vi "CaseMonitor__slk_mt.vi"() -> ()   [LabVIEW 2012, in "Lazyboots Menu Tool.lvlib"]
doc: "This VI is the core of <b>Case Monitor</b> function, and will be called by corresponding menu launcher."
uses:
  Library/Lazyboots Menu Tool.lvlib
  Private/CaseMonitor/Class/TreeView/TreeView__slk_mt.lvclass
  Private/CaseMonitor/Class/CaseModel/CaseModel__slk_mt.lvclass
  Private/CaseMonitor/Class/DatatypeAdapter/DatatypeAdapter__slk_mt.lvclass
  <vilib>/Utility/config.llb/NI_LVConfig.lvlib
panel:
  in  "Case Frames Tree":string(tree)
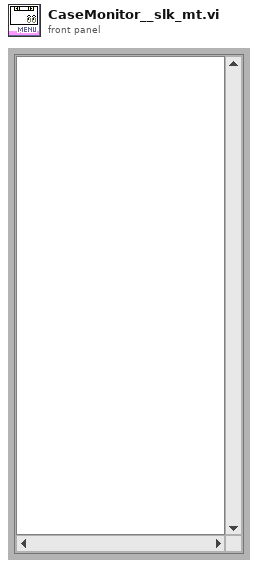
[diagram p1: front panel]
types:
  T1 = enum32{"Invalid", "Standard", "Closed", "Hidden", "Minimized", "Maximized"}
  T2 = cluster{"ItemTag":string, "OldFrame":string, "NewFrame":string}
  T3 = cluster{"Application Refnum":refnum<vi>, "VI Name":string}
  T4 = typedef "NI_LVConfig.lvlib/Config Data RefNum.ctl" = refnum<k1>
  T5 = typedef "Lazyboots Menu Tool.lvlib/TypeDef_CaseMonitorConfigure__slk_mt.ctl" = cluster{"Parent Symbol":string}
  T6 = typedef "LVPoint32TypeDef.ctl" = cluster{"Horizontal":i32, "Vertical":i32}
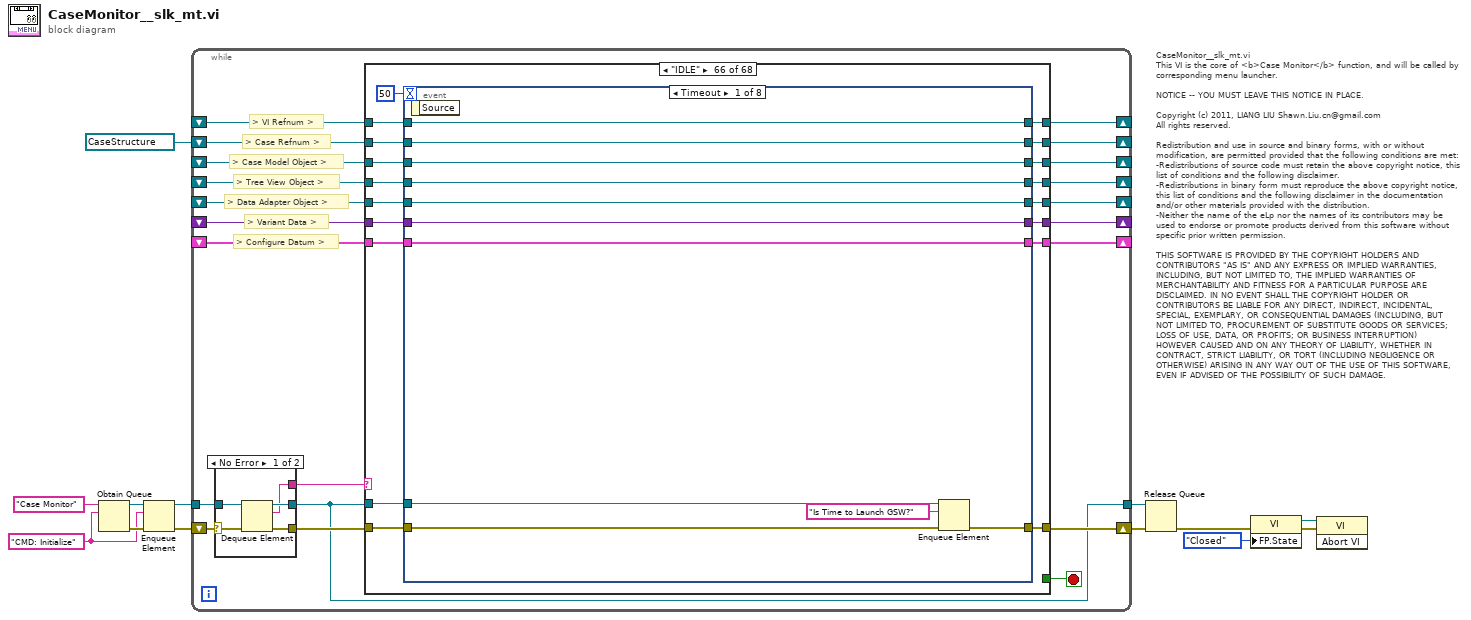
[diagram p0: block diagram]
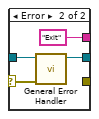
[diagram p2: hidden frame]
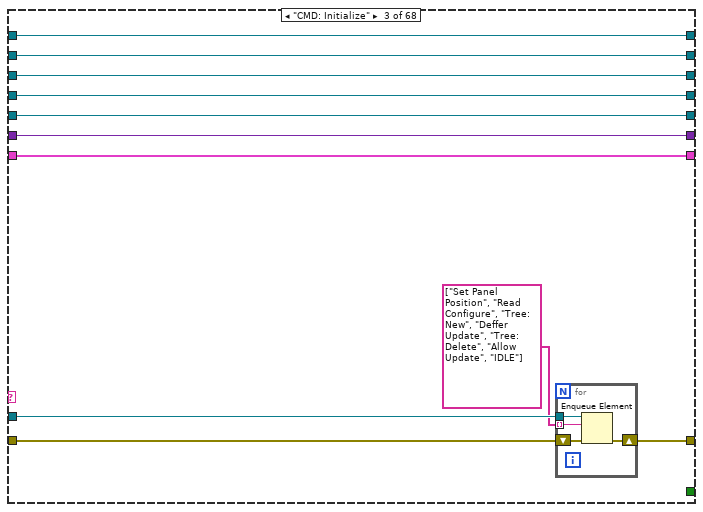
[diagram p5: hidden frame]
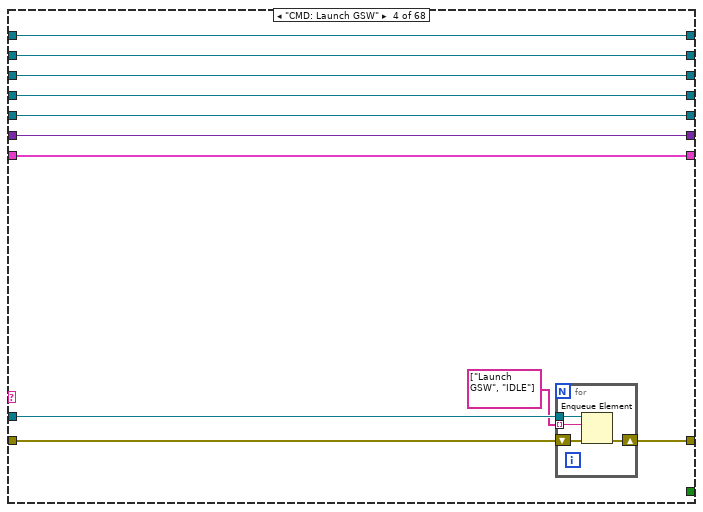
[diagram p6: hidden frame]
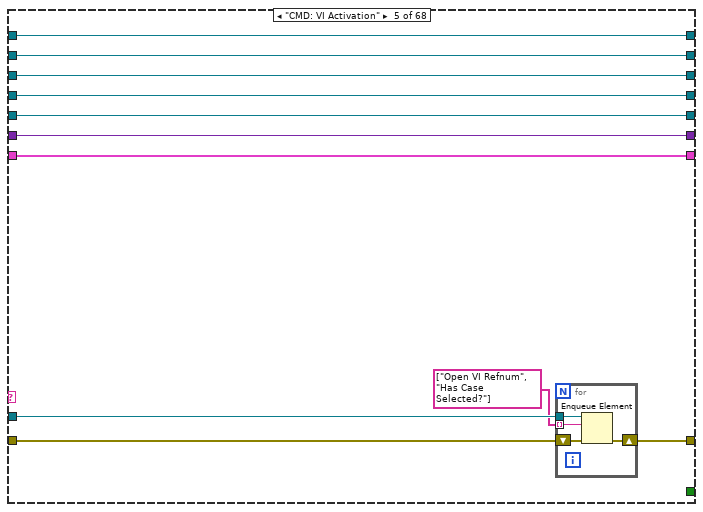
[diagram p7: hidden frame]
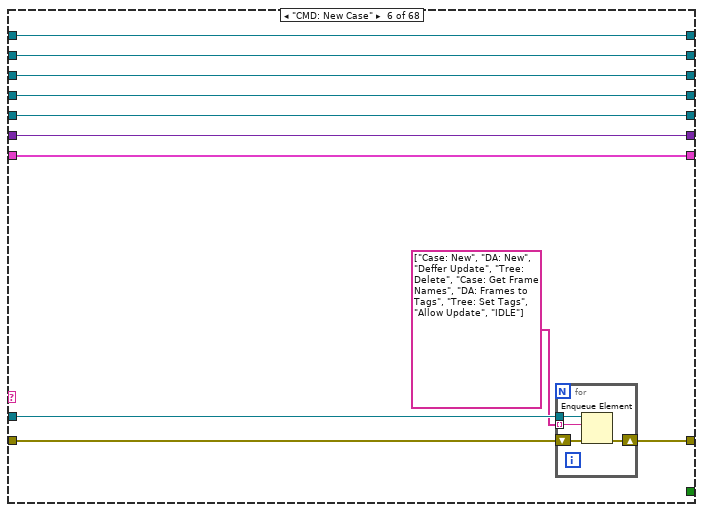
[diagram p8: hidden frame]
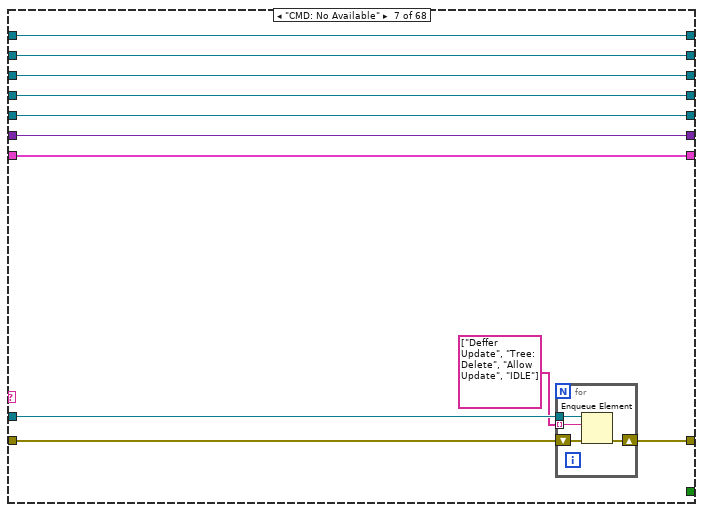
[diagram p9: hidden frame]
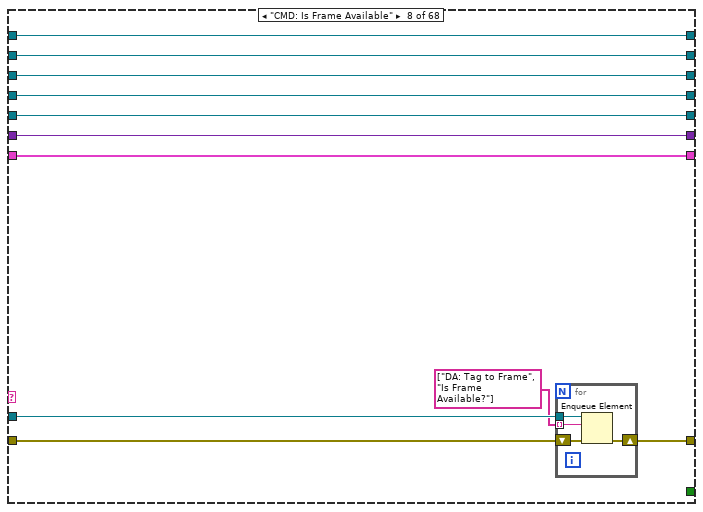
[diagram p10: hidden frame]
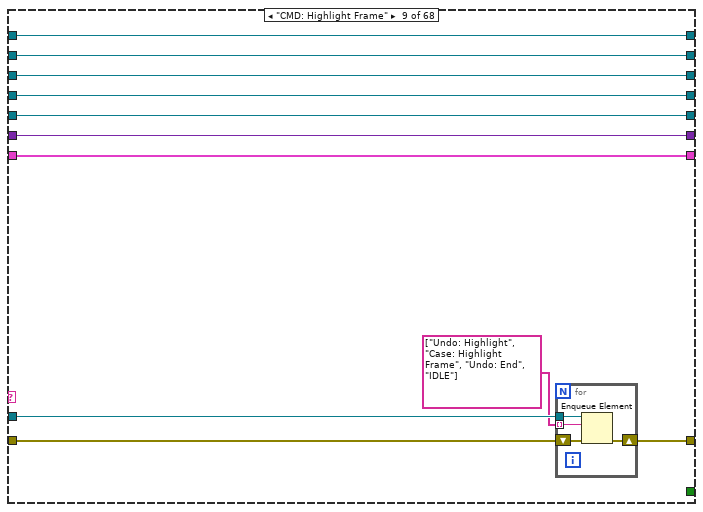
[diagram p11: hidden frame]
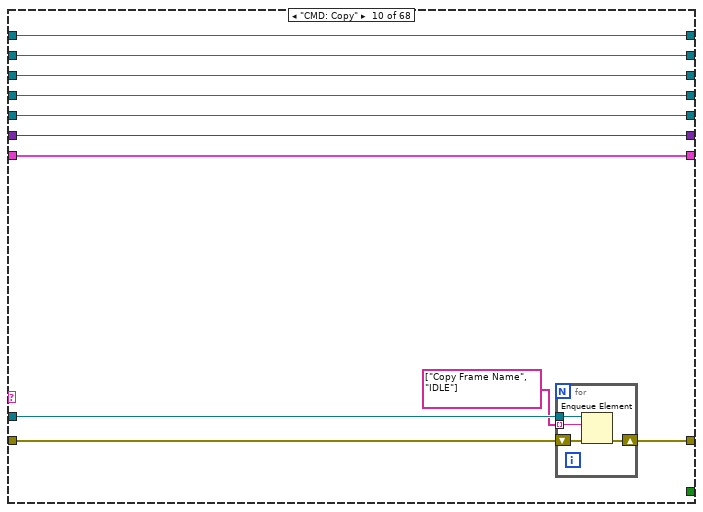
[diagram p12: hidden frame]
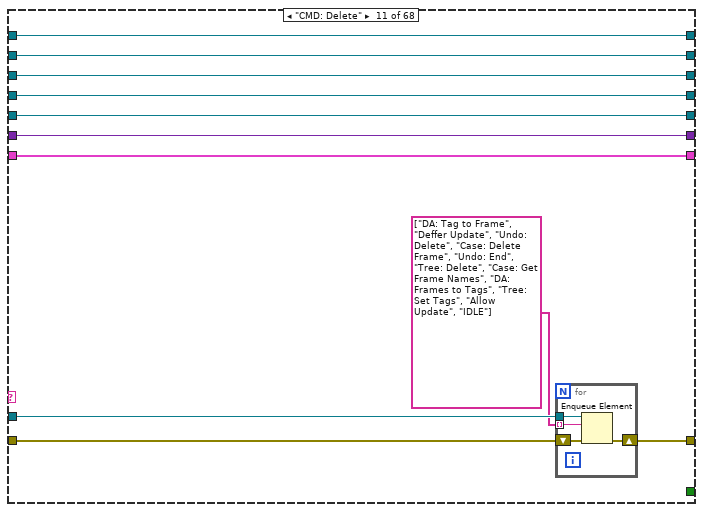
[diagram p13: hidden frame]
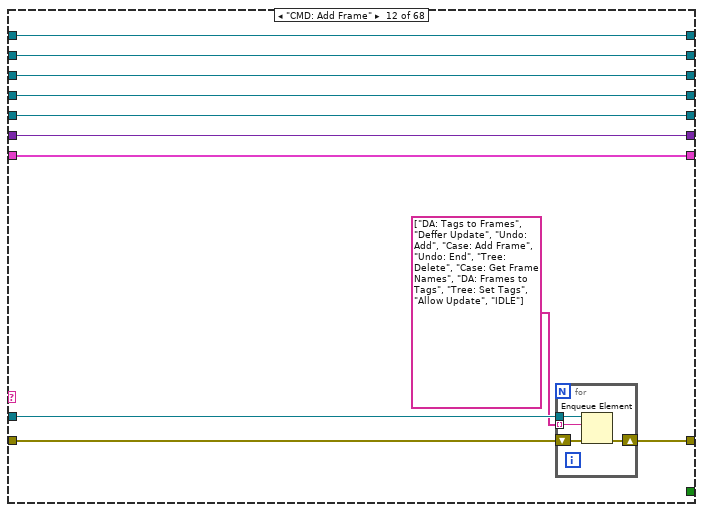
[diagram p14: hidden frame]
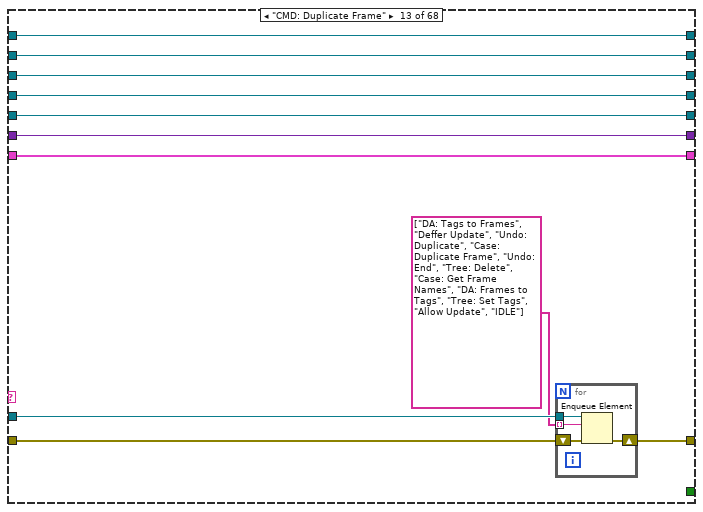
[diagram p15: hidden frame]
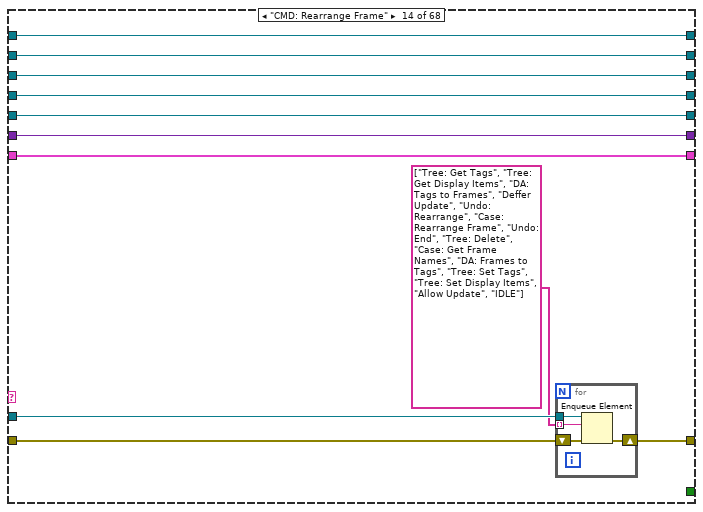
[diagram p16: hidden frame]
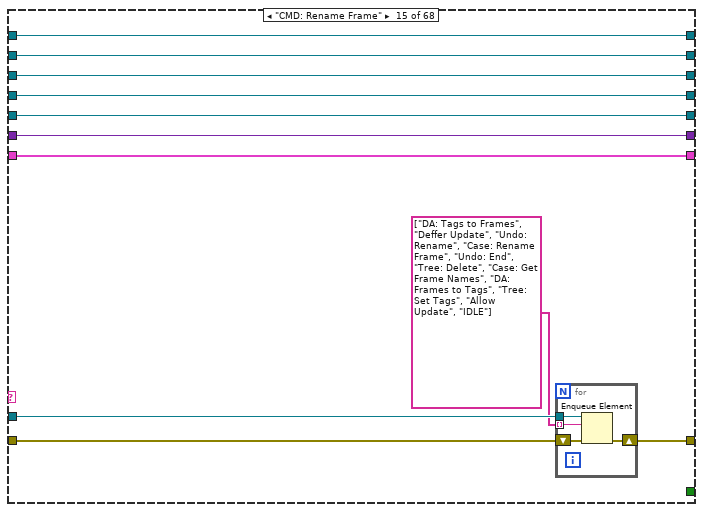
[diagram p17: hidden frame]
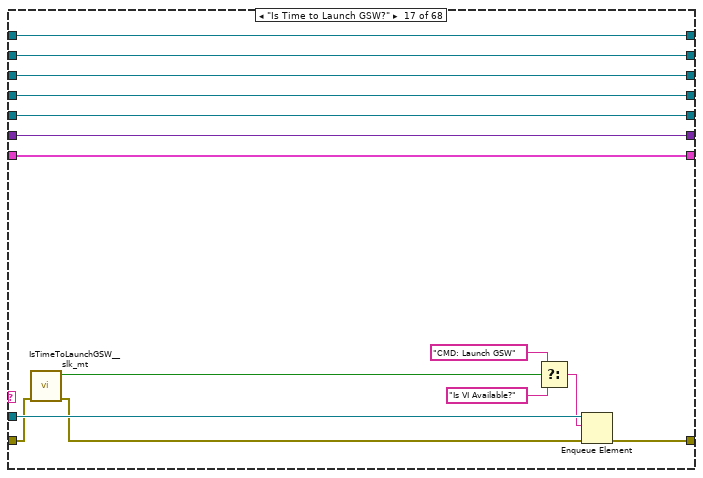
[diagram p19: hidden frame]
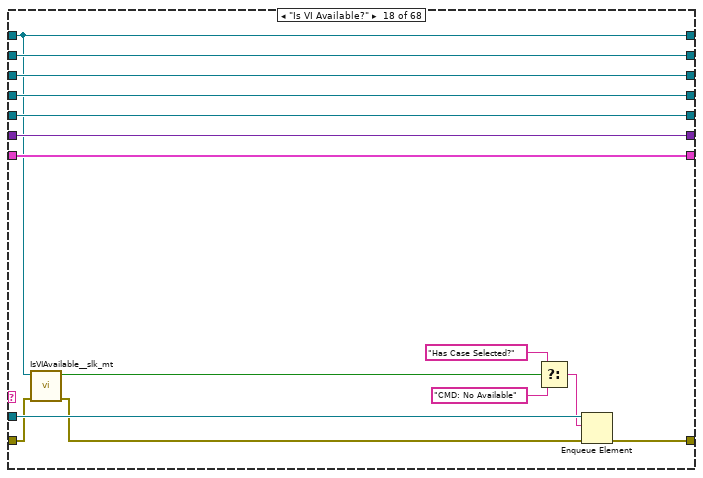
[diagram p20: hidden frame]
diagram:
  w6 = "CMD: Initialize" ("State")
  # "CaseMonitor__slk_mt.vi\nThis VI is the core of <b>Case Monitor</b> function, and will be called by corresponding menu launcher.\n\nNOTICE -- YOU MUST LEAVE THIS NOTICE IN PLACE.\n\nCopyright (c) 2011, LIANG LIU Shawn.Liu.cn@gmail.com\nAll rights reserved.\n\nRedistribution and use in source and binary forms, with or without modification, are permitted provided that the following conditions are met:\n-Redistributions of source code must retain the above copyright notice, this list of conditions and the following disclaimer.\n-Redistributions in binary form must reproduce the above copyright notice, this list of conditions and the following disclaimer in the documentation and/or other materials provided with the distribution.\n-Neither the name of the eLp nor the names of its contributors may be used to endorse or promote products derived from this software without specific prior written permission.\n\nTHIS SOFTWARE IS PROVIDED BY THE COPYRIGHT HOLDERS AND CONTRIBUTORS \"AS IS\" AND ANY EXPRESS OR IMPLIED WARRANTIES, INCLUDING, BUT NOT LIMITED TO, THE IMPLIED WARRANTIES OF MERCHANTABILITY AND FITNESS FOR A PARTICULAR PURPOSE ARE DISCLAIMED. IN NO EVENT SHALL THE COPYRIGHT HOLDER OR CONTRIBUTORS BE LIABLE FOR ANY DIRECT, INDIRECT, INCIDENTAL, SPECIAL, EXEMPLARY, OR CONSEQUENTIAL DAMAGES (INCLUDING, BUT NOT LIMITED TO, PROCUREMENT OF SUBSTITUTE GOODS OR SERVICES; LOSS OF USE, DATA, OR PROFITS; OR BUSINESS INTERRUPTION) HOWEVER CAUSED AND ON ANY THEORY OF LIABILITY, WHETHER IN CONTRACT, STRICT LIABILITY, OR TORT (INCLUDING NEGLIGENCE OR OTHERWISE) ARISING IN ANY WAY OUT OF THE USE OF THIS SOFTWARE, EVEN IF ADVISED OF THE POSSIBILITY OF SUCH DAMAGE."
  n1 = Obtain Queue(name (unnamed)="Case Monitor" ("Queue Name"), element data type=w6) -> (queue out=w12:refnum<queue>, error out=w11:errorcluster)  [unwired: 3 in, 1 out]
  n2 = Enqueue Element(queue=w12, element=w6, error in (no error)=w11) -> (queue out=w8:refnum<queue>, error out=w7:errorcluster)  [unwired: 2 out]
  n3 = while {
    tunnel: w8 -> [w33]
    shift-right: [w31] -> w9
    shift-left: w7 -> [w34]
    shift-right: [w20] -> _
    shift-left: _ -> [w14]
    shift-right: [w27] -> _
    shift-left: refnum<vi> refnum ("case refnum out") -> [w30]
    shift-right: [w28] -> _
    shift-left: _ -> [w29]
    tunnel: [w26] -> w10
    shift-right: [w22] -> _
    shift-left: _ -> [w24]
    shift-right: [w21] -> _
    shift-left: _ -> [w23]
    shift-right: [w17] -> _
    shift-left: _ -> [w18]
    shift-right: [w15] -> _
    shift-left: _ -> [w16]
    stop <- w25 stop-if-true
    # "> Configure Datum >"
    # "> Variant Data >"
    # "> Data Adapter Object >"
    # "> Case Model Object >"
    # "> Tree View Object >"
    # "> Case Refnum >"
    # "> VI Refnum >"
    n4 = case shown="No Error" w34 {
      selector: w34 -> [w38 w42]
      tunnel: w33 -> [w39 w41]
      tunnel: [w37 _] -> w32
      tunnel: [w36 w41] -> w26
      tunnel: [w35 "Exit" ("State")] -> w19
      frame No Error {
        n5 = Dequeue Element(queue=w39, error in (no error)=w38) -> (queue out=w36:refnum<queue>, element=w35:string, error out=w37:errorcluster)  [unwired: 2 out]
      }
      frame Error {
        n6 = call <vilib>:"General Error Handler.vi"("error in (no error)"=w42) -> ()  [unwired: 2 in, 13 out]
      }
    }
    n7 = case shown="\"IDLE\"" w19 {
      tunnel: w32 -> [w50 w58 w67 w82 w97 w112 w127 w142 w157 w172 w187 w202 w217 w232 w247 w261 w271 w286 w302 w317 w335 w365 w386 w413 w429 w432 w448 w464 w478 w486 w498 w514 w518 w534 w544 w553 w566 w569 w581 w591 w604 w613 w623 w633 w645 w660 w675 w690 w702 w714 w722 w731 w745 w759 w773 w787 w795 w799 w809 w819 w829 w839 w849 w859 w872 w889 w1076 w1085]
      tunnel: [w50 w58 w64 w79 w94 w109 w124 w139 w154 w169 w184 w199 w214 w229 w244 w261 w273 w288 w305 w320 w338 w368 w389 w416 w429 w433 w446 w459 w470 w483 w495 w505 w525 w534 w540 w549 w564 w575 w585 w595 w604 w611 w614 w630 w643 w658 w673 w688 w700 w712 w722 w729 w743 w757 w771 w785 w795 w798 w808 w818 w828 w838 w848 w858 w872 w888 w1076 w1085] -> w31
      tunnel: w26 -> [_ _ w63 w78 w93 w108 w123 w138 w153 w168 w183 w198 w213 w228 w243 _ w272 w287 w304 w319 w337 w367 w388 w415 _ _ _ _ _ _ _ _ w524 _ _ _ _ _ _ _ _ _ _ _ _ _ _ _ _ _ _ _ _ _ _ _ _ _ _ _ _ _ _ _ _ w890 _ _]
      tunnel: w14 -> [w45 w53 w62 w77 w92 w107 w122 w137 w152 w167 w182 w197 w212 w227 w242 w256 w264 w277 w303 w318 w336 w366 w387 w414 w424 w441 w450 w457 _ w484 w496 w512 w523 w529 w537 w548 w563 w574 w584 w594 w599 w610 w620 w629 w642 w657 w672 w687 w699 w711 w717 w728 w742 w756 w770 w784 w790 w797 w807 w817 w827 w837 w847 w857 w867 w887 w1071 w1079]
      tunnel: [w45 w53 w62 w77 w92 w107 w122 w137 w152 w167 w182 w197 w212 w227 w242 w256 w264 w277 w303 w318 w336 w366 w387 w414 w424 w441 w450 w457 w472 w484 w496 w512 w523 w529 w537 w548 w563 w574 w584 w594 w599 w610 w620 w629 w642 w657 w672 w687 w699 w711 w717 w728 w742 w756 w770 w784 w790 w797 w807 w817 w827 w837 w847 w857 w867 w877 w1071 w1079] -> w20
      tunnel: w30 -> [w48 w56 w68 w83 w98 w113 w128 w143 w158 w173 w188 w203 w218 w233 w248 w259 w266 w279 w293 w311 w325 w361 w384 w411 w427 w444 w453 w462 w476 w489 w501 w513 w522 w532 w542 w551 w565 w576 w586 w596 w602 w606 w617 w632 w644 w659 w674 w689 w701 w713 w720 w730 w744 w758 w772 w786 w793 w804 w814 w824 w834 w844 w854 w863 w870 w886 w1074 w1083]
      tunnel: w29 -> [w49 w57 w69 w84 w99 w114 w129 w144 w159 w174 w189 w204 w219 w234 w249 w260 w276 w291 w308 w323 w341 w371 w376 w417 w428 w445 w454 w463 w477 w490 w502 w510 w526 w533 w543 w552 w562 w573 w583 w593 w603 _ w615 w625 w635 w651 w666 w681 w692 w705 w721 w726 w740 w754 w768 w782 w794 w805 w815 w825 w835 w845 w855 w864 w871 w885 w1075 w1084]
      tunnel: [w49 w57 w69 w84 w99 w114 w129 w144 w159 w174 w189 w204 w219 w234 w249 w260 w276 w291 w308 w323 w341 w371 w376 w417 w428 w445 w454 w463 w477 w490 w502 w510 w526 w533 w543 w552 w562 w573 w583 w593 w603 w608 w615 w625 w635 w651 w666 w681 w692 w705 w721 w726 w740 w754 w768 w782 w794 w805 w815 w825 w835 w845 w855 w864 w871 w884 w1075 w1084] -> w28
      tunnel: [w48 w56 w68 w83 w98 w113 w128 w143 w158 w173 w188 w203 w218 w233 w248 w259 w266 w279 w293 w311 w327 w361 w384 w411 w427 w444 w453 w462 w476 w489 w501 w513 w522 w532 w542 w551 w565 w576 w586 w596 w602 w606 w617 w632 w644 w659 w674 w689 w701 w713 w720 w730 w744 w758 w772 w786 w793 w804 w814 w824 w834 w844 w854 w863 w870 w883 w1074 w1083] -> w27
      tunnel: [_ _ _ _ _ _ _ _ _ _ _ _ _ _ _ _ _ _ _ _ _ _ _ _ _ _ _ _ _ _ _ _ _ _ _ _ _ _ _ _ _ _ _ _ _ _ _ _ _ _ _ _ _ _ _ _ _ _ _ _ _ _ _ _ _ _ _ TRUE] -> w25
      tunnel: w24 -> [w46 w54 w65 w80 w95 w110 w125 w140 w155 w170 w185 w200 w215 w230 w245 w257 w274 w289 w306 w321 w339 w369 w383 w399 w425 w442 w451 w460 w474 w487 w499 w511 w521 w530 _ w546 w557 w571 w579 w589 w600 w609 w619 w628 w641 w656 w671 w686 w698 w710 w718 w727 w741 w755 w769 w783 w791 w802 w812 w822 w832 w842 w852 w861 w868 w881 w1072 w1081]
      tunnel: w23 -> [w47 w55 w66 w81 w96 w111 w126 w141 w156 w171 w186 w201 w216 w231 w246 w258 w275 w290 w307 w322 w340 w370 w382 w398 w426 w443 w452 w461 w475 w488 w500 w509 w520 w531 w541 w550 w561 w572 w582 w592 w601 w612 w622 w631 w640 w655 w670 w685 w697 w709 w719 _ w739 w753 w767 w781 w792 w803 w813 w823 w833 w843 w853 w862 w869 w880 w1073 w1082]
      tunnel: [w46 w54 w65 w80 w95 w110 w125 w140 w155 w170 w185 w200 w215 w230 w245 w257 w274 w289 w306 w321 w339 w369 w383 w399 w425 w442 w451 w460 w474 w487 w499 w511 w521 w530 w538 w546 w557 w571 w578 w588 w600 w609 w619 w628 w641 w656 w671 w686 w698 w710 w718 w727 w741 w755 w769 w783 w791 w802 w812 w822 w832 w842 w852 w861 w868 w879 w1072 w1081] -> w22
      tunnel: [w47 w55 w66 w81 w96 w111 w126 w141 w156 w171 w186 w201 w216 w231 w246 w258 w275 w290 w307 w322 w340 w370 w382 w398 w426 w443 w452 w461 w475 w488 w500 w509 w520 w531 w541 w550 w561 w572 w582 w592 w601 w612 w622 w631 w640 w655 w670 w685 w697 w709 w719 w725 w739 w753 w767 w781 w792 w803 w813 w823 w833 w843 w853 w862 w869 w878 w1073 w1082] -> w21
      tunnel: w18 -> [w44 w52 w60 w75 w90 w105 w120 w135 w150 w165 w180 w195 w210 w225 w240 w255 w265 w281 _ w310 w330 w348 w378 w410 w423 w440 w449 w456 w466 w480 w492 w507 w519 w528 w536 w547 w556 _ w580 w590 w598 w607 w618 _ w636 w653 w668 w683 w693 w706 w716 w724 w736 w750 w764 w778 w789 w801 w811 w821 w831 w841 w851 w860 w866 w875 w1070 w1078]
      tunnel: [w44 w52 w60 w75 w90 w105 w120 w135 w150 w165 w180 w195 w210 w225 w240 w255 w265 w281 w295 w310 w330 w349 w378 w405 w423 w440 w449 w456 w466 w480 w492 w507 w519 w528 w536 w547 w556 w568 w580 w590 w598 w607 w618 w626 w636 w653 w668 w683 w693 w706 w716 w724 w733 w747 w761 w775 w789 w801 w811 w821 w831 w841 w851 w860 w866 w876 w1070 w1078] -> w17
      tunnel: w16 -> [w43 w51 w59 w74 w89 w104 w119 w134 w149 w164 w179 w194 w209 w224 w239 w254 w263 w280 w292 w309 w324 w342 w379 w390 w422 _ w447 w455 w465 w479 w491 w503 w515 w527 w535 w545 w555 w567 w577 w587 w597 w605 w616 w624 w634 w646 w661 w676 w691 w703 w715 w723 w732 w746 w760 w774 w788 w796 w806 w816 w826 w836 w846 w856 w865 w874 w1069 w1077]
      tunnel: [w43 w51 w59 w74 w89 w104 w119 w134 w149 w164 w179 w194 w209 w224 w239 w254 w263 w280 w292 w309 w324 w342 w379 w390 w422 w430 w447 w455 w465 w479 w491 w503 w515 w527 w535 w545 w555 w567 w577 w587 w597 w605 w616 w624 w634 w646 w661 w676 w691 w703 w715 w723 w732 w746 w760 w774 w788 w796 w806 w816 w826 w836 w846 w856 w865 w873 w1069 w1077] -> w15
      frame Default {
      }
      frame "----Command----" {
      }
      frame "CMD: Initialize" {
        n8 = for {
          tunnel: w63 -> [w71]
          shift-right: [w72] -> w64
          shift-left: w67 -> [w73]
          tunnel: string[] ["Set Panel Position", "Read Configure", "Tree: New", "Deffer Update", "Tree: Delete", "Allow Update", "IDLE"] -> [w70] mode=indexing
          n9 = Enqueue Element(queue=w71, element=w70, error in (no error)=w73) -> (error out=w72:errorcluster)  [unwired: 1 in, 2 out]
        }
      }
      frame "CMD: Launch GSW" {
        n10 = for {
          tunnel: w78 -> [w86]
          shift-right: [w87] -> w79
          shift-left: w82 -> [w88]
          tunnel: string[] ["Launch GSW", "IDLE"] -> [w85] mode=indexing
          n11 = Enqueue Element(queue=w86, element=w85, error in (no error)=w88) -> (error out=w87:errorcluster)  [unwired: 1 in, 2 out]
        }
      }
      frame "CMD: VI Activation" {
        n12 = for {
          tunnel: w93 -> [w101]
          shift-right: [w102] -> w94
          shift-left: w97 -> [w103]
          tunnel: string[] ["Open VI Refnum", "Has Case Selected?"] -> [w100] mode=indexing
          n13 = Enqueue Element(queue=w101, element=w100, error in (no error)=w103) -> (error out=w102:errorcluster)  [unwired: 1 in, 2 out]
        }
      }
      frame "CMD: New Case" {
        n14 = for {
          tunnel: w108 -> [w116]
          shift-right: [w117] -> w109
          shift-left: w112 -> [w118]
          tunnel: string[] ["Case: New", "DA: New", "Deffer Update", "Tree: Delete", "Case: Get Frame Names", "DA: Frames to Tags", "Tree: Set Tags", "Allow Update", "IDLE"] -> [w115] mode=indexing
          n15 = Enqueue Element(queue=w116, element=w115, error in (no error)=w118) -> (error out=w117:errorcluster)  [unwired: 1 in, 2 out]
        }
      }
      frame "CMD: No Available" {
        n16 = for {
          tunnel: w123 -> [w131]
          shift-right: [w132] -> w124
          shift-left: w127 -> [w133]
          tunnel: string[] ["Deffer Update", "Tree: Delete", "Allow Update", "IDLE"] -> [w130] mode=indexing
          n17 = Enqueue Element(queue=w131, element=w130, error in (no error)=w133) -> (error out=w132:errorcluster)  [unwired: 1 in, 2 out]
        }
      }
      frame "CMD: Is Frame Available" {
        n18 = for {
          tunnel: w138 -> [w146]
          shift-right: [w147] -> w139
          shift-left: w142 -> [w148]
          tunnel: string[] ["DA: Tag to Frame", "Is Frame Available?"] -> [w145] mode=indexing
          n19 = Enqueue Element(queue=w146, element=w145, error in (no error)=w148) -> (error out=w147:errorcluster)  [unwired: 1 in, 2 out]
        }
      }
      frame "CMD: Highlight Frame" {
        n20 = for {
          tunnel: w153 -> [w161]
          shift-right: [w162] -> w154
          shift-left: w157 -> [w163]
          tunnel: string[] ["Undo: Highlight", "Case: Highlight Frame", "Undo: End", "IDLE"] -> [w160] mode=indexing
          n21 = Enqueue Element(queue=w161, element=w160, error in (no error)=w163) -> (error out=w162:errorcluster)  [unwired: 1 in, 2 out]
        }
      }
      frame "CMD: Copy" {
        n22 = for {
          tunnel: w168 -> [w176]
          shift-right: [w177] -> w169
          shift-left: w172 -> [w178]
          tunnel: string[] ["Copy Frame Name", "IDLE"] -> [w175] mode=indexing
          n23 = Enqueue Element(queue=w176, element=w175, error in (no error)=w178) -> (error out=w177:errorcluster)  [unwired: 1 in, 2 out]
        }
      }
      frame "CMD: Delete" {
        n24 = for {
          tunnel: w183 -> [w191]
          shift-right: [w192] -> w184
          shift-left: w187 -> [w193]
          tunnel: string[] ["DA: Tag to Frame", "Deffer Update", "Undo: Delete", "Case: Delete Frame", "Undo: End", "Tree: Delete", "Case: Get Frame Names", "DA: Frames to Tags", "Tree: Set Tags", "Allow Update", "IDLE"] -> [w190] mode=indexing
          n25 = Enqueue Element(queue=w191, element=w190, error in (no error)=w193) -> (error out=w192:errorcluster)  [unwired: 1 in, 2 out]
        }
      }
      frame "CMD: Add Frame" {
        n26 = for {
          tunnel: w198 -> [w206]
          shift-right: [w207] -> w199
          shift-left: w202 -> [w208]
          tunnel: string[] ["DA: Tags to Frames", "Deffer Update", "Undo: Add", "Case: Add Frame", "Undo: End", "Tree: Delete", "Case: Get Frame Names", "DA: Frames to Tags", "Tree: Set Tags", "Allow Update", "IDLE"] -> [w205] mode=indexing
          n27 = Enqueue Element(queue=w206, element=w205, error in (no error)=w208) -> (error out=w207:errorcluster)  [unwired: 1 in, 2 out]
        }
      }
      frame "CMD: Duplicate Frame" {
        n28 = for {
          tunnel: w213 -> [w221]
          shift-right: [w222] -> w214
          shift-left: w217 -> [w223]
          tunnel: string[] ["DA: Tags to Frames", "Deffer Update", "Undo: Duplicate", "Case: Duplicate Frame", "Undo: End", "Tree: Delete", "Case: Get Frame Names", "DA: Frames to Tags", "Tree: Set Tags", "Allow Update", "IDLE"] -> [w220] mode=indexing
          n29 = Enqueue Element(queue=w221, element=w220, error in (no error)=w223) -> (error out=w222:errorcluster)  [unwired: 1 in, 2 out]
        }
      }
      frame "CMD: Rearrange Frame" {
        n30 = for {
          tunnel: w228 -> [w236]
          shift-right: [w237] -> w229
          shift-left: w232 -> [w238]
          tunnel: string[] ["Tree: Get Tags", "Tree: Get Display Items", "DA: Tags to Frames", "Deffer Update", "Undo: Rearrange", "Case: Rearrange Frame", "Undo: End", "Tree: Delete", "Case: Get Frame Names", "DA: Frames to Tags", "Tree: Set Tags", "Tree: Set Display Items", "Allow Update", "IDLE"] -> [w235] mode=indexing
          n31 = Enqueue Element(queue=w236, element=w235, error in (no error)=w238) -> (error out=w237:errorcluster)  [unwired: 1 in, 2 out]
        }
      }
      frame "CMD: Rename Frame" {
        n32 = for {
          tunnel: w243 -> [w251]
          shift-right: [w252] -> w244
          shift-left: w247 -> [w253]
          tunnel: string[] ["DA: Tags to Frames", "Deffer Update", "Undo: Rename", "Case: Rename Frame", "Undo: End", "Tree: Delete", "Case: Get Frame Names", "DA: Frames to Tags", "Tree: Set Tags", "Allow Update", "IDLE"] -> [w250] mode=indexing
          n33 = Enqueue Element(queue=w251, element=w250, error in (no error)=w253) -> (error out=w252:errorcluster)  [unwired: 1 in, 2 out]
        }
      }
      frame "----Query----" {
      }
      frame "Is Time to Launch GSW?" {
        n34 = call "IsTimeToLaunchGSW__slk_mt.vi"("error in (no error)"=w271) -> ("error out"=w270:errorcluster, "ready?"=w262:bool)  [unwired: 9 in]
        n35 = Select(t="CMD: Launch GSW" ("State"), s=w262, f="Is VI Available?" ("State")) -> (s? t:f=w269:string)
        n36 = Enqueue Element(queue=w272, element=w269, error in (no error)=w270) -> (error out=w273:errorcluster)  [unwired: 1 in, 2 out]
      }
      frame "Is VI Available?" {
        n37 = call "IsVIAvailable__slk_mt.vi"("error in (no error)"=w286, "vi refnum in"=w277) -> ("error out"=w285:errorcluster, "available?"=w278:bool)  [unwired: 8 in]
        n38 = Select(t="Has Case Selected?" ("State"), s=w278, f="CMD: No Available" ("State")) -> (s? t:f=w284:string)
        n39 = Enqueue Element(queue=w287, element=w284, error in (no error)=w285) -> (error out=w288:errorcluster)  [unwired: 1 in, 2 out]
      }
      frame "Has Case Selected?" {
        n40 = call "GetCaseRefnum__slk_mt.vi"("error in (no error)"=w302, "vi refnum in"=w303) -> ("error out"=w301:errorcluster, "not found?"=w297:bool, "case refnum out"=w294:refnum<vi>)  [unwired: 7 in]
        n41 = Select(t=w293, s=w297, f=w294) -> (s? t:f=w296:refnum<vi>)
        n42 = To Variant(anything=w296) -> (Variant=w295:variant)
        n43 = Select(t="Is Case Available?" ("State"), s=w297, f="New Case?" ("State")) -> (s? t:f=w300:string)
        n44 = Enqueue Element(queue=w304, element=w300, error in (no error)=w301) -> (error out=w305:errorcluster)  [unwired: 1 in, 2 out]
      }
      frame "Is Case Available?" {
        n45 = call "IsCaseAvailable__slk_mt.vi"("error in (no error)"=w317, "case refnum in"=w311) -> ("error out"=w316:errorcluster, "available?"=w313:bool)  [unwired: 8 in]
        n46 = Select(t="New Case?" ("State"), s=w313, f="CMD: No Available" ("State")) -> (s? t:f=w315:string)
        n47 = Enqueue Element(queue=w319, element=w315, error in (no error)=w316) -> (error out=w320:errorcluster)  [unwired: 1 in, 2 out]
      }
      frame "New Case?" {
        n48 = Variant To Data(error in=w335, type=refnum<vi> refnum ("case refnum out"), Variant=w330) -> (data=w326:refnum<vi>, error out=w334:errorcluster)
        n49 = Equal?(x=w325, y=w326) -> (x = y?=w328:bool)
        n50 = Select(t=w325, s=w328, f=w326) -> (s? t:f=w327:refnum<vi>)
        n51 = Select(t="IDLE" ("State"), s=w328, f="CMD: New Case" ("State")) -> (s? t:f=w333:string)
        n52 = Enqueue Element(queue=w337, element=w333, error in (no error)=w334) -> (error out=w338:errorcluster)  [unwired: 1 in, 2 out]
      }
      frame "User Prompt?" {
        n53 = Variant To Data(error in=w365, type=cluster{"ItemTag":string, "Tag":string} {"ItemTag"="", "Tag"=""} ("cluster"), Variant=w348) -> (data=w354:cluster{"ItemTag":string, "Tag":string}, error out=w355:errorcluster)
        n54 = Unbundle By Name(w354) -> ("ItemTag"=w357:string, "Tag"=w346:string)
        n55 = Equal?(x="Rename Frame...", y=w357) -> (x = y?=w359:bool)
        n56 = Select(t=w346, s=w359, f="") -> (s? t:f=w345:string)
        n57 = call "UserPrompt__slk_mt.vi"("error in (no error)"=w355, "new frame name in (\"\")"=w345) -> ("error out"=w353:errorcluster, "ok?"=w343:bool, "new frame name out"=w344:string)  [unwired: 7 in]
        n58 = Bundle By Name(cluster=T2 {"ItemTag"="", "OldFrame"="", "NewFrame"=""}, "ItemTag"=w357, "OldFrame"=w346, "NewFrame"=w344) -> (w351:T2)
        n59 = Not(x=w343) -> (.not. x?=w347:bool)
        n60 = To Variant(anything=w351) -> (Variant=w350:variant)
        n61 = Select(t=w348, s=w347, f=w350) -> (s? t:f=w349:variant)
        n62 = Select(t="IDLE" ("State"), s=w347, f="Is Repeat Tag?" ("State")) -> (s? t:f=w364:string)
        n63 = Enqueue Element(queue=w367, element=w364, error in (no error)=w353) -> (error out=w368:errorcluster)  [unwired: 1 in, 2 out]
      }
      frame "Is Frame Available?" {
        n64 = Variant To Data(error in=w386, type="", Variant=w378) -> (data=w375:string, error out=w374:errorcluster)
        n65 = call "IsFrameAvailable__slk_mt.vi"("error in (no error)"=w374, "frame name"=w375, "case model in"=w376) -> ("error out"=w372:errorcluster, "available?"=w373:bool)  [unwired: 6 in, 1 out]
        n66 = Select(t="CMD: Highlight Frame" ("State"), s=w373, f="CMD: New Case" ("State")) -> (s? t:f=w385:string)
        n67 = Enqueue Element(queue=w388, element=w385, error in (no error)=w372) -> (error out=w389:errorcluster)  [unwired: 1 in, 2 out]
      }
      frame "Is Repeat Tag?" {
        n68 = Variant To Data(error in=w413, type=T2 {"ItemTag"="", "OldFrame"="", "NewFrame"=""}, Variant=w410) -> (data=w397:T2, error out=w402:errorcluster)
        n69 = Unbundle By Name(w397) -> ("NewFrame"=w391:string, "OldFrame"=w394:string, "ItemTag"=w396:string)
        n70 = call-dynamic "FrameToTag(scalar)__slk_mt.vi"("error in (no error)"=w402, "frame"=w391, "adapter in"=w398) -> ("error out"=w403:errorcluster, "tag"=w400:string)  [unwired: 6 in, 1 out]
        n71 = call "IsRepeatTag__slk_mt.vi"("error in (no error)"=w403, "tag"=w400, "tree view in"=w399) -> ("error out"=w401:errorcluster, "repeat?"=w404:bool)  [unwired: 6 in, 1 out]
        n72 = Bundle By Name(cluster=cluster{"NewFrame":string, "OldFrame":string} {"NewFrame"="", "OldFrame"=""}, "NewFrame"=w391, "OldFrame"=w394) -> (w407:cluster{"NewFrame":string, "OldFrame":string})
        n73 = Not(x=w404) -> (.not. x?=w392:bool)
        n74 = Cluster To Array(cluster=w407) -> (array=w406:string[])
        n75 = To Variant(anything=w406) -> (Variant=w405:variant)
        n76 = case shown="\"Add Frame After...\"" w396 {
          tunnel: ["IDLE" ("State") "CMD: Add Frame" ("State") "CMD: Duplicate Frame" ("State") "CMD: Rename Frame" ("State")] -> w395
          frame Default {
          }
          frame "Add Frame After..." {
          }
          frame "Duplicate Frame After..." {
          }
          frame "Rename Frame..." {
          }
        }
        n77 = Select(t=w395, s=w392, f="Error Message" ("State")) -> (s? t:f=w412:string)
        n78 = Enqueue Element(queue=w415, element=w412, error in (no error)=w401) -> (error out=w416:errorcluster)  [unwired: 1 in, 2 out]
      }
      frame "----Monitor----" {
      }
      frame "Read Configure" {
        n79 = Current VI's Path() -> (path=w435:path)
        n80 = Build Path(base path=w435, name or relative path=path "../../Configure/SLK Menu Tool.ini") -> (appended path=w434:path)
        n81 = call <vilib>:"Open Config Data.vi"("error in (no error)"=w432, "configuration file path"=w434) -> ("error out"=w438:errorcluster, "refnum"=w439:T4)  [unwired: 7 in, 1 out]
        n82 = call "ReadCaseMonitor__slk_mt.vi"("error in (no error)"=w438, "refnum in"=w439) -> ("error out"=w437:errorcluster, "case monitor configure"=w430:T5, "refnum out"=w436:T4)  [unwired: 7 in]
        n83 = call <vilib>:"Close Config Data.vi"("error in (no error)"=w437, "refnum"=w436) -> ("error out"=w433:errorcluster)  [unwired: 8 in, 1 out]
      }
      frame "Launch GSW" {
        n84 = call "LaunchGSW__slk_mt.vi"("error in (no error)"=w448) -> ("error out"=w446:errorcluster)  [unwired: 10 in]
      }
      frame "Set Panel Position" {
        n85 = control-ref of="This VI"() -> (w458:refnum<vi>)
        n86 = call "SetPanelPosition__slk_mt.vi"("error in (no error)"=w464, "vi refnum in"=w458) -> ("error out"=w459:errorcluster)  [unwired: 9 in]
      }
      frame "Open VI Refnum" {
        n87 = Variant To Data(error in=w478, type=T3 {"Application Refnum"=refnum, "VI Name"=""} ("VI Activation"), Variant=w466) -> (data=w467:T3, error out=w471:errorcluster)
        n88 = Unbundle(w467) -> ("Application Refnum"=w469:refnum<vi>, "VI Name"=w468:string)
        n89 = Open VI Reference(application reference (local)=w469, vi path=w468, error in (no error)=w471) -> (vi reference=w472:refnum<vi>, error out=w470:errorcluster)  [unwired: 3 in]
      }
      frame "Deffer Update" {
        n90 = property on="Property Node" class="VI"(error in=w486) -> (error out=w482:errorcluster, "Panel"=w485:refnum<vi>)  [unwired: 1 in, 1 out]
        n91 = property on="Property Node" class="Pnl"(reference=w485, error in=w482, "DeferPanUpdts"=TRUE ("Defer Panel Updates")) -> (error out=w483:errorcluster)  [unwired: 1 out]
      }
      frame "Allow Update" {
        n92 = property on="Property Node" class="VI"(error in=w498) -> (error out=w494:errorcluster, "Panel"=w497:refnum<vi>)  [unwired: 1 in, 1 out]
        n93 = property on="Property Node" class="Pnl"(reference=w497, error in=w494, "DeferPanUpdts"=FALSE ("Defer Panel Updates")) -> (error out=w495:errorcluster)  [unwired: 1 out]
      }
      frame "Copy Frame Name" {
        n94 = Variant To Data(error in=w514, type="", Variant=w507) -> (data=w504:string, error out=w506:errorcluster)
        n95 = invoke class="App" method="Clipboard.Write"(error in=w506, "Param 0"=w504) -> (error out=w505:errorcluster)  [unwired: 2 in, 3 out]
      }
      frame "Error Message" {
        n96 = call "Message__slk_mt.vi"("error in (no error)"=w518) -> ("error out"=w517:errorcluster)  [unwired: 10 in]
        n97 = Enqueue Element(queue=w524, element="IDLE", error in (no error)=w517) -> (error out=w525:errorcluster)  [unwired: 1 in, 2 out]
      }
      frame "----Tree----" {
      }
      frame "Tree: New" {
        n98 = control-ref of="Case Frames Tree"() -> (w539:refnum<vi>)
        n99 = call "New__slk_mt.vi"("error in (no error)"=w544, "tree refnum in"=w539) -> ("error out"=w540:errorcluster, "tree view out"=w538:refnum<class "TreeView__slk_mt.lvclass">)  [unwired: 8 in]
      }
      frame "Tree: Delete" {
        n100 = call "DeleteTree__slk_mt.vi"("error in (no error)"=w553, "tree view in"=w546) -> ("error out"=w549:errorcluster)  [unwired: 8 in, 1 out]
      }
      frame "Tree: Set Tags" {
        n101 = Variant To Data(error in=w566, type=string[] [], Variant=w556) -> (data=w558:string[], error out=w560:errorcluster)
        n102 = Unbundle(w555) -> ("Parent Symbol"=w554:string)
        n103 = call "SetTreeTags__slk_mt.vi"("error in (no error)"=w560, "parents symbol (-)"=w554, "tags in"=w558, "tree view in"=w557) -> ("error out"=w564:errorcluster)  [unwired: 6 in, 1 out]
      }
      frame "Tree: Get Tags" {
        n104 = call "GetTreeTags__slk_mt.vi"("error in (no error)"=w569, "tree view in"=w571) -> ("error out"=w575:errorcluster, "tags"=w570:string[])  [unwired: 7 in, 1 out]
        n105 = To Variant(anything=w570) -> (Variant=w568:variant)
      }
      frame "Tree: Get Display Items" {
        n106 = call "GetDisplayItems__slk_mt.vi"("error in (no error)"=w581, "tree view in"=w579) -> ("error out"=w585:errorcluster, "tree view out"=w578:refnum<class "TreeView__slk_mt.lvclass">)  [unwired: 8 in]
      }
      frame "Tree: Set Display Items" {
        n107 = call "SetDisplayItems__slk_mt.vi"("error in (no error)"=w591, "tree view in"=w589) -> ("error out"=w595:errorcluster, "tree view out"=w588:refnum<class "TreeView__slk_mt.lvclass">)  [unwired: 8 in]
      }
      frame "----Case----" {
      }
      frame "Case: New" {
        n108 = call "New__slk_mt.vi"("error in (no error)"=w613, "case refnum in"=w606) -> ("error out"=w611:errorcluster, "case model out"=w608:refnum<class "CaseModel__slk_mt.lvclass">)  [unwired: 8 in]
      }
      frame "Case: Close" {
        n109 = call "Close__slk_mt.vi"("error in (no error)"=w623, "case model in"=w615) -> ("error out"=w621:errorcluster)  [unwired: 9 in]
        n110 = call <vilib>:"Clear Errors.vi"("error in (no error)"=w621) -> ("error out"=w614:errorcluster)  [unwired: 5 in, 1 out]
      }
      frame "Case: Get Frame Names" {
        n111 = call "GetFrameNames__slk_mt.vi"("error in (no error)"=w633, "case model in"=w625) -> ("error out"=w630:errorcluster, "frame names"=w627:string[])  [unwired: 7 in, 1 out]
        n112 = To Variant(anything=w627) -> (Variant=w626:variant)
      }
      frame "Case: Highlight Frame" {
        n113 = Variant To Data(error in=w645, type="", Variant=w636) -> (data=w637:string, error out=w639:errorcluster)
        n114 = call "ShowAndHighlightFrame__slk_mt.vi"("error in (no error)"=w639, "frame name"=w637, "case model in"=w635) -> ("error out"=w643:errorcluster)  [unwired: 7 in, 1 out]
      }
      frame "Case: Add Frame" {
        n115 = Variant To Data(error in=w660, type=string[] [], Variant=w653) -> (data=w650:string[], error out=w654:errorcluster)
        n116 = Array To Cluster(array=w650) -> (cluster=w649:cluster{"[0]":string, "[1]":string})
        n117 = Unbundle(w649) -> ("[0]"=w648:string, "[1]"=w647:string)
        n118 = call "AddFrame__slk_mt.vi"("error in (no error)"=w654, "add after frame name"=w647, "new frame name"=w648, "case model in"=w651) -> ("error out"=w658:errorcluster)  [unwired: 6 in, 1 out]
      }
      frame "Case: Duplicate Frame" {
        n119 = Variant To Data(error in=w675, type=string[] [], Variant=w668) -> (data=w665:string[], error out=w669:errorcluster)
        n120 = Array To Cluster(array=w665) -> (cluster=w664:cluster{"[0]":string, "[1]":string})
        n121 = Unbundle(w664) -> ("[0]"=w663:string, "[1]"=w662:string)
        n122 = call "DuplicateFrame__slk_mt.vi"("error in (no error)"=w669, "source frame name"=w662, "new frame name"=w663, "case model in"=w666) -> ("error out"=w673:errorcluster)  [unwired: 6 in, 1 out]
      }
      frame "Case: Rename Frame" {
        n123 = Variant To Data(error in=w690, type=string[] [], Variant=w683) -> (data=w680:string[], error out=w684:errorcluster)
        n124 = Array To Cluster(array=w680) -> (cluster=w679:cluster{"[0]":string, "[1]":string})
        n125 = Unbundle(w679) -> ("[0]"=w678:string, "[1]"=w677:string)
        n126 = call "RenameFrame__slk_mt.vi"("error in (no error)"=w684, "old frame name"=w677, "new frame name"=w678, "case model in"=w681) -> ("error out"=w688:errorcluster)  [unwired: 6 in, 1 out]
      }
      frame "Case: Delete Frame" {
        n127 = Variant To Data(error in=w702, type="", Variant=w693) -> (data=w694:string, error out=w696:errorcluster)
        n128 = call "DeleteFrame__slk_mt.vi"("error in (no error)"=w696, "frame name"=w694, "case model in"=w692) -> ("error out"=w700:errorcluster)  [unwired: 7 in, 1 out]
      }
      frame "Case: Rearrange Frame" {
        n129 = Variant To Data(error in=w714, type=string[] [], Variant=w706) -> (data=w707:string[], error out=w708:errorcluster)
        n130 = call "RearrangeFrameByNames__slk_mt.vi"("error in (no error)"=w708, "frame names"=w707, "case model in"=w705) -> ("error out"=w712:errorcluster)  [unwired: 7 in, 1 out]
      }
      frame "----Data Adapter----" {
      }
      frame "DA: New" {
        n131 = call "New__slk_mt.vi"("error in (no error)"=w731, "case model in"=w726) -> ("error out"=w729:errorcluster, "adapter out"=w725:refnum<class "DatatypeAdapter__slk_mt.lvclass">)  [unwired: 8 in]
      }
      frame "DA: Frame to Tag" {
        n132 = Variant To Data(error in=w745, type="", Variant=w736) -> (data=w734:string, error out=w737:errorcluster)
        n133 = call-dynamic "FrameToTag(scalar)__slk_mt.vi"("error in (no error)"=w737, "frame"=w734, "adapter in"=w739) -> ("error out"=w743:errorcluster, "tag"=w738:string)  [unwired: 6 in, 1 out]
        n134 = To Variant(anything=w738) -> (Variant=w733:variant)
      }
      frame "DA: Frames to Tags" {
        n135 = Variant To Data(error in=w759, type=string[] [], Variant=w750) -> (data=w748:string[], error out=w751:errorcluster)
        n136 = call-dynamic "FrameToTag(array)__slk_mt.vi"("error in (no error)"=w751, "frames"=w748, "adapter in"=w753) -> ("error out"=w757:errorcluster, "tags"=w752:string[])  [unwired: 6 in, 1 out]
        n137 = To Variant(anything=w752) -> (Variant=w747:variant)
      }
      frame "DA: Tag to Frame" {
        n138 = Variant To Data(error in=w773, type="", Variant=w764) -> (data=w762:string, error out=w765:errorcluster)
        n139 = call-dynamic "TagToFrame(scalar)__slk_mt.vi"("error in (no error)"=w765, "tag"=w762, "adapter in"=w767) -> ("error out"=w771:errorcluster, "frame"=w766:string)  [unwired: 6 in, 1 out]
        n140 = To Variant(anything=w766) -> (Variant=w761:variant)
      }
      frame "DA: Tags to Frames" {
        n141 = Variant To Data(error in=w787, type=string[] [], Variant=w778) -> (data=w776:string[], error out=w779:errorcluster)
        n142 = call-dynamic "TagToFrame(array)__slk_mt.vi"("error in (no error)"=w779, "tags"=w776, "adapter in"=w781) -> ("error out"=w785:errorcluster, "frames"=w780:string[])  [unwired: 6 in, 1 out]
        n143 = To Variant(anything=w780) -> (Variant=w775:variant)
      }
      frame "----Undo----" {
      }
      frame "Undo: Delete" {
        n144 = invoke class="VI" method="Transaction.Begin Undo"(reference=w797, error in=w799, "Name"="CaseMonitor.Delete__slk_mt") -> (error out=w798:errorcluster)  [unwired: 1 in, 3 out]
      }
      frame "Undo: Add" {
        n145 = invoke class="VI" method="Transaction.Begin Undo"(reference=w807, error in=w809, "Name"="CaseMonitor.Add__slk_mt") -> (error out=w808:errorcluster)  [unwired: 1 in, 3 out]
      }
      frame "Undo: Duplicate" {
        n146 = invoke class="VI" method="Transaction.Begin Undo"(reference=w817, error in=w819, "Name"="CaseMonitor.Duplicate__slk_mt") -> (error out=w818:errorcluster)  [unwired: 1 in, 3 out]
      }
      frame "Undo: Rename" {
        n147 = invoke class="VI" method="Transaction.Begin Undo"(reference=w827, error in=w829, "Name"="CaseMonitor.Rename__slk_mt") -> (error out=w828:errorcluster)  [unwired: 1 in, 3 out]
      }
      frame "Undo: Rearrange" {
        n148 = invoke class="VI" method="Transaction.Begin Undo"(reference=w837, error in=w839, "Name"="CaseMonitor.Rearrange__slk_mt") -> (error out=w838:errorcluster)  [unwired: 1 in, 3 out]
      }
      frame "Undo: Highlight" {
        n149 = invoke class="VI" method="Transaction.Begin Undo"(reference=w847, error in=w849, "Name"="CaseMonitor.Highlight__slk_mt") -> (error out=w848:errorcluster)  [unwired: 1 in, 3 out]
      }
      frame "Undo: End" {
        n150 = invoke class="VI" method="Transaction.End Undo"(reference=w857, error in=w859) -> (error out=w858:errorcluster)  [unwired: 1 in, 2 out]
      }
      frame "----Event----" {
      }
      frame "IDLE" {
        n151 = event shown="[0] Timeout" {
          selector: _ -> [_ _ _ _ _ _ _ _]
          dyn-events: _ -> [_ _ _ _ _ _ _ _]
          timeout: 50 -> [_ _ _ _ _ _ _ _]
          tunnel: w890 -> [w897 w919 w929 w956 w987 w1009 w1045 w1064]
          tunnel: w889 -> [w893 w914 w931 w958 w989 w1011 w1043 w1062]
          tunnel: [w901 w920 w930 w957 w988 w1010 w1046 w1065] -> w888
          tunnel: w887 -> [w900 w925 w937 w962 w992 w1014 w1049 w1068]
          tunnel: [w900 w925 w937 w962 w992 w1014 w1049 w1068] -> w877
          tunnel: w886 -> [w899 w924 w936 w961 w991 w1013 w1048 w1067]
          tunnel: w885 -> [w898 w923 w935 w960 w970 w1008 w1044 w1063]
          tunnel: [w898 w923 w935 w960 w970 w1008 w1044 w1063] -> w884
          tunnel: [w899 w924 w936 w961 w991 w1013 w1048 w1067] -> w883
          tunnel: w881 -> [w896 w922 w934 w954 w969 w1007 w1041 w1061]
          tunnel: w880 -> [w895 w921 w933 w959 w990 w1012 w1047 w1066]
          tunnel: [w896 w922 w934 w954 w969 w1007 w1040 w1052] -> w879
          tunnel: [w895 w921 w933 w959 w990 w1012 w1047 w1066] -> w878
          tunnel: [w891 w910 w927 w953 w984 w1001 w1039 w1060] -> w876
          tunnel: w875 -> [w891 _ w927 w945 w984 w1002 w1039 w1060]
          tunnel: w874 -> [w892 w907 w926 w942 w993 w1015 w1037 w1050]
          tunnel: [w892 w907 w926 w942 w993 w1015 w1037 w1050] -> w873
          event Timeout {
            n152 = event-data() -> ()  [unwired: 2 out]
            n153 = Enqueue Element(queue=w897, element="Is Time to Launch GSW?", error in (no error)=w893) -> (error out=w901:errorcluster)  [unwired: 3 out]
          }
          event VI Activation {
            n154 = event-data() -> ("VIAppRef"=w917:refnum<vi>, "VIName"=w905:string)  [unwired: 1 out]
            n155 = control-ref of="This VI"() -> (w915:refnum<vi>)
            n156 = property class="VI"(reference=w915, error in=w914) -> (error out=w913:errorcluster, "Name"=w911:string)  [unwired: 1 out]
            n157 = Not Equal?(x=w905, y=w911) -> (x != y?=w906:bool)
            n158 = Bundle By Name(cluster=T3 {"Application Refnum"=refnum, "VI Name"=""} ("VI Activation"), "Application Refnum"=w917, "VI Name"=w905) -> (w916:T3)
            n159 = Not Equal?(x="GettingStartedWindow.lvlibp:GSW_Main.vi", y=w905) -> (x != y?=w902:bool)
            n160 = And(x=w902, y=w906) -> (x .and. y?=w904:bool)
            n161 = To Variant(anything=w916) -> (Variant=w910:variant)
            n162 = Select(t="CMD: VI Activation" ("State"), s=w904, f="IDLE" ("State")) -> (s? t:f=w912:string)
            n163 = Enqueue Element(queue=w919, element=w912, error in (no error)=w913) -> (error out=w920:errorcluster)  [unwired: 1 in, 2 out]
          }
          event Panel Close? {
            n164 = event-data() -> ()  [unwired: 2 out]
            n165 = for {
              tunnel: w929 -> [w939]
              shift-right: [w940] -> w930
              shift-left: w931 -> [w941]
              tunnel: string[] ["Tree: Delete", "Exit"] -> [w938] mode=indexing
              n166 = Enqueue Element(queue=w939, element=w938, error in (no error)=w941) -> (error out=w940:errorcluster)  [unwired: 1 in, 2 out]
            }
            n167 = event-data("Discard?"=TRUE) -> ()  [unwired: 1 in, 1 out]
          }
          event "Case Frames Tree": Double Click {
            n168 = event-data() -> ("Coords"=w955:T6)  [unwired: 1 out]
            n169 = call "GetTagByCoords__slk_mt.vi"("error in (no error)"=w958, "coordinates"=w955, "tree view in"=w954) -> ("error out"=w948:errorcluster, "tag"=w946:string, "tree view out"=w949:refnum<class "TreeView__slk_mt.lvclass">)  [unwired: 6 in]
            n170 = To Variant(anything=w946) -> (Variant=w944:variant)
            n171 = call "IsRepeatTag__slk_mt.vi"("error in (no error)"=w948, "tag"=w946, "tree view in"=w949) -> ("error out"=w947:errorcluster, "repeat?"=w943:bool)  [unwired: 6 in, 1 out]
            n172 = Select(t=w944, s=w943, f=w945) -> (s? t:f=w953:variant)
            n173 = Select(t="CMD: Is Frame Available" ("element"), s=w943, f="IDLE" ("element")) -> (s? t:f=w950:string)
            n174 = Enqueue Element(queue=w956, element=w950, error in (no error)=w947) -> (error out=w957:errorcluster)  [unwired: 1 in, 2 out]
          }
          event "Case Frames Tree": Shortcut Menu Activation? {
            w981 = "Delete Frame" ("item name")
            n175 = event-data() -> ("MenuRef"=w972:refnum<k9>, "Coords"=w985:T6)  [unwired: 1 out]
            n176 = call "GetTagByCoords__slk_mt.vi"("error in (no error)"=w989, "coordinates"=w985, "tree view in"=w969) -> ("error out"=w974:errorcluster, "tag"=w966:string, "tree view out"=w967:refnum<class "TreeView__slk_mt.lvclass">)  [unwired: 6 in]
            n177 = call "SetActiveTag__slk_mt.vi"("error in (no error)"=w974, "tag"=w966, "tree view in"=w967) -> ("error out"=w964:errorcluster, "duplicated tag"=w965:string)  [unwired: 6 in, 1 out]
            n178 = call "GetFrameNames__slk_mt.vi"("error in (no error)"=w964, "case model in"=w970) -> ("error out"=w963:errorcluster, "frame names"=w977:string[])  [unwired: 7 in, 1 out]
            n179 = Empty String/Path?(string/path=w965) -> (empty?=w976:bool)
            n180 = Array Size(array=w977) -> (size(s)=w968:i32)
            n181 = Not(x=w976) -> (.not. x?=w983:bool)
            n182 = Greater?(x=w968, y=1) -> (0:w978:bool)
            n183 = for {
              tunnel: string[] ["Add Frame After...", "Duplicate Frame After...", "Rename Frame...", "Copy Frame Name"] -> [w995] mode=indexing
              shift-right: [w998] -> w979
              shift-left: w963 -> [w997]
              tunnel: w983 -> [w996]
              shift-right: [w994] -> w980
              shift-left: w972 -> [w999]
              n184 = Set Menu Item Info(7:w995, 8:w997, 9:w996, 10:w995, 11:w999) -> (0:w998:errorcluster, 3:w994:refnum<k9>)  [unwired: 2 in]
            }
            n185 = Compound Arithmetic op=AND(w983, w978) -> (w982:bool)
            n186 = Set Menu Item Info(7:w981, 8:w979, 9:w982, 10:w981, 11:w980) -> (0:w973:errorcluster)  [unwired: 2 in, 1 out]
            n187 = Enqueue Element(queue=w987, element="IDLE", error in (no error)=w973) -> (error out=w988:errorcluster)  [unwired: 1 in, 2 out]
            n188 = event-data() -> ()  [unwired: 2 in, 1 out]
          }
          event "Case Frames Tree": Shortcut Menu Selection (User) {
            n189 = event-data() -> ("ItemTag"=w1005:string, "Coords"=w1006:T6)  [unwired: 2 out]
            n190 = call "GetTagByCoords__slk_mt.vi"("error in (no error)"=w1011, "coordinates"=w1006, "tree view in"=w1007) -> ("error out"=w1004:errorcluster, "tag"=w1003:string)  [unwired: 6 in, 1 out]
            n191 = in-place {
              in-place-border: w1005 -> [w1020]
              in-place-border: w1003 -> [w1019]
              in-place-border: [w1016] -> w1000
              n192 = in-place-match #1(w1002) -> (w1018:variant)
              n193 = case shown="\"Refresh List\"" w1020 {
                selector: w1020 -> [_ _ w1030 _ _]
                tunnel: w1019 -> [_ _ w1026 w1033 w1036]
                tunnel: ["IDLE" ("State") "CMD: New Case" ("State") "User Prompt?" ("State") "CMD: Delete" ("State") "CMD: Copy" ("State")] -> w1016
                tunnel: w1018 -> [w1022 w1024 _ _ _]
                tunnel: [w1022 w1024 w1027 w1032 w1035] -> w1017
                frame Default {
                }
                frame "Refresh List" {
                }
                frame "Add Frame After...", "Duplicate Frame After...", "Rename Frame..." {
                  n194 = Bundle(cluster=cluster{"ItemTag":string, "Tag":string} {"ItemTag"="", "Tag"=""}, "ItemTag"=w1030, "Tag"=w1026) -> (w1029:cluster{"ItemTag":string, "Tag":string})
                  n195 = To Variant(anything=w1029) -> (Variant=w1027:variant)
                }
                frame "Delete Frame" {
                  n196 = To Variant(anything=w1033) -> (Variant=w1032:variant)
                }
                frame "Copy Frame Name" {
                  n197 = To Variant(anything=w1036) -> (Variant=w1035:variant)
                }
              }
              n198 = in-place-match #1(w1017) -> (w1001:variant)
            }
            n199 = Enqueue Element(queue=w1009, element=w1000, error in (no error)=w1004) -> (error out=w1010:errorcluster)  [unwired: 1 in, 2 out]
          }
          event "Case Frames Tree": Drag Starting {
            n200 = event-data() -> ()  [unwired: 2 out]
            n201 = call "SetDragInfo__slk_mt.vi"("error in (no error)"=w1043, "tree view in"=w1041) -> ("error out"=w1042:errorcluster, "tree view out"=w1040:refnum<class "TreeView__slk_mt.lvclass">)  [unwired: 8 in]
            n202 = Enqueue Element(queue=w1045, element="IDLE", error in (no error)=w1042) -> (error out=w1046:errorcluster)  [unwired: 1 in, 2 out]
          }
          event "Case Frames Tree": Drop {
            n203 = event-data() -> ("Coords"=w1058:T6)  [unwired: 1 out]
            n204 = call "GetTagByCoords__slk_mt.vi"("error in (no error)"=w1062, "coordinates"=w1058, "tree view in"=w1061) -> ("error out"=w1055:errorcluster, "tag"=w1056:string, "tree view out"=w1057:refnum<class "TreeView__slk_mt.lvclass">)  [unwired: 6 in]
            n205 = call "SetDropInfo__slk_mt.vi"("error in (no error)"=w1055, "drop tag"=w1056, "tree view in"=w1057) -> ("error out"=w1053:errorcluster, "tree view out"=w1054:refnum<class "TreeView__slk_mt.lvclass">)  [unwired: 7 in]
            n206 = call "DropTag__slk_mt.vi"("error in (no error)"=w1053, "tree view in"=w1054) -> ("error out"=w1051:errorcluster, "tree view out"=w1052:refnum<class "TreeView__slk_mt.lvclass">)  [unwired: 8 in]
            n207 = Enqueue Element(queue=w1064, element="CMD: Rearrange Frame", error in (no error)=w1051) -> (error out=w1065:errorcluster)  [unwired: 1 in, 2 out]
            n208 = event-data() -> ()  [unwired: 2 in, 1 out]
          }
        }
      }
      frame "----Exit----" {
      }
      frame "Exit" {
      }
    }
  }
  n209 = Release Queue(queue=w10, error in (no error)=w9) -> (error out=w3:errorcluster)  [unwired: 3 out]
  n210 = property class="VI"(error in=w3, "FP.State"=T1."Closed" ("Front Panel Window:State")) -> (reference out=w2:refnum<vi>, error out=w1:errorcluster)  [unwired: 1 in]
  n211 = invoke class="VI" method="Abort VI"(reference=w2, error in=w1) -> ()  [unwired: 1 in, 3 out]
